vi "AddTwoNumbers - Shell.vi"(10 "Numeric 2":dbl, 11 "Numeric":dbl) -> (3 "Numeric 4":dbl)   [LabVIEW 2009]
panel:
  in  "Numeric 3":dbl
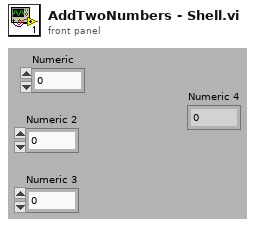
[diagram p1: front panel]
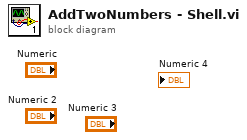
[diagram p0: block diagram]
diagram:
